vi "Read UI Constants.vi"(8 "Error In":errorcluster, 11 "refnum":T2) -> (0 "Error Out":errorcluster, 2 "output cluster":T1, 3 "refnum out":T2)   [LabVIEW 2015]
uses:
  <vilib>/Utility/config.llb/Config Data RefNum.ctl
  controls/MHL Configuration.ctl
  Boiler System Globals.vi
  <vilib>/Utility/config.llb/Read Key (Double).vi
  <vilib>/Utility/config.llb/NI_LVConfig.lvlib
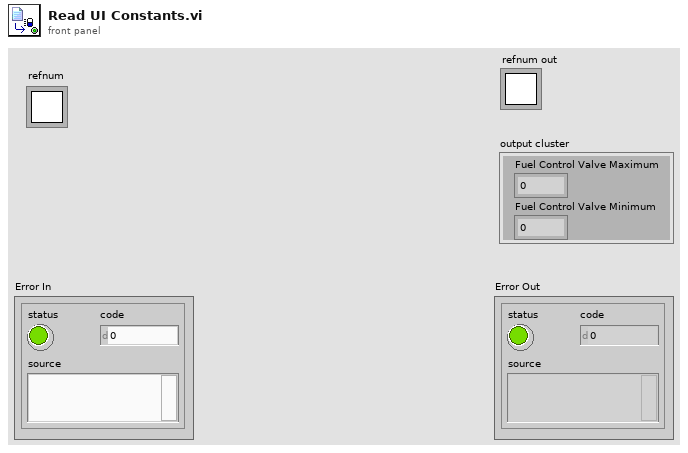
[diagram p1: front panel]
types:
  T1 = typedef "MHL Configuration.ctl" = cluster{"Fuel Control Valve Maximum":dbl, "Fuel Control Valve Minimum":dbl}
  T2 = typedef "NI_LVConfig.lvlib/Config Data RefNum.ctl" = refnum<k1>
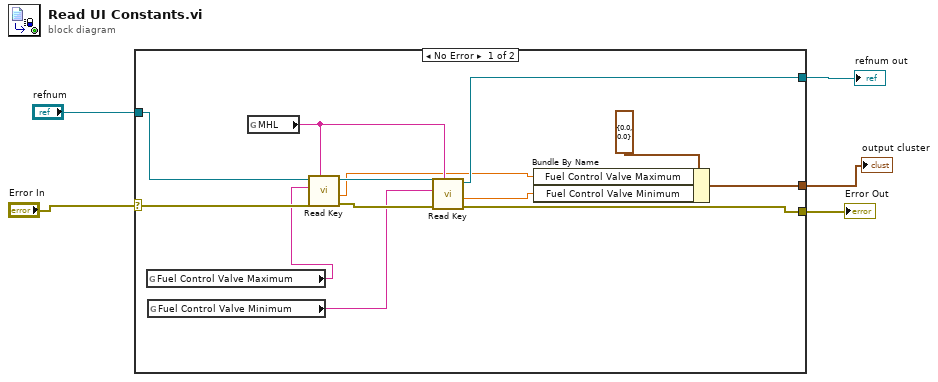
[diagram p0: block diagram]
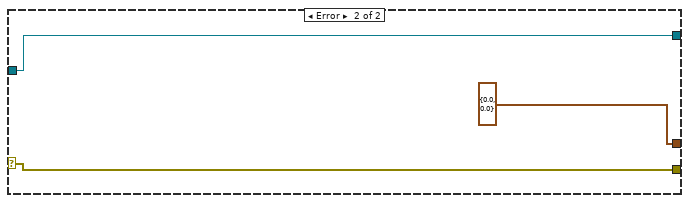
[diagram p2: hidden frame]
diagram:
  n1 = case shown="No Error" "Error In" {
    selector: "Error In" -> [w18 w20]
    tunnel: [w16 w20] -> w4
    tunnel: "refnum" -> [w12 w21]
    tunnel: [w10 w21] -> w2
    tunnel: [w6 T1 {"Fuel Control Valve Maximum"=0.0, "Fuel Control Valve Minimum"=0.0} ("MHL Configuration")] -> w1
    frame No Error {
      n2 = global read "Boiler System Globals.vi" "Fuel Control Valve Maximum"() -> (w14:string)
      n3 = global read "Boiler System Globals.vi" "Fuel Control Valve Minimum"() -> (w13:string)
      n4 = global read "Boiler System Globals.vi" "MHL"() -> (w15:string)
      n5 = call-poly <vilib>:"Read Key.vi"("section"=w15, "error in (no error)"=w18, "key"=w14, "refnum"=w12) -> ("error out"=w17:errorcluster, "value"=w8:dbl, "refnum out"=w11:T2)  [unwired: 4 in, 1 out]
      n6 = call-poly <vilib>:"Read Key.vi"("section"=w15, "error in (no error)"=w17, "key"=w13, "refnum"=w11) -> ("error out"=w16:errorcluster, "value"=w7:dbl, "refnum out"=w10:T2)  [unwired: 4 in, 1 out]
      n7 = Bundle By Name(cluster=T1 {"Fuel Control Valve Maximum"=0.0, "Fuel Control Valve Minimum"=0.0} ("MHL Configuration"), "Fuel Control Valve Maximum"=w8, "Fuel Control Valve Minimum"=w7) -> (w6:T1)
    }
    frame Error {
    }
  }
  "Error Out" <- w4
  "refnum out" <- w2
  "output cluster" <- w1
